vi "Burning.vi"(8 "error in (no error)":errorcluster, 9 "TimeOut(s)":dbl, 10 "burnFilePath":path=path "D:/Project/Tymphany/LT_UpgradeFlash/HDMI Board/LT FW  Files/LT9611 UXC/lt9611uxc_fw.bin", 11 "LT_UpgradeFlash in":refnum<class "LT_UpgradeFlash.lvclass">) -> (0 "error out":errorcluster, 1 "resultStr":string, 2 "ActionResult":bool, 3 "LT_UpgradeFlash out":refnum<class "LT_UpgradeFlash.lvclass">)   [LabVIEW 2017, in "LT_UpgradeFlash.lvclass"]
uses:
  LT_UpgradeFlash.lvclass
  D:/Project/Tymphany/LT_UpgradeFlash/New_Lib/LT_UpgradeFlash_dll/LT_UpgradeFlash_dll/bin/Debug/LT_UpgradeFlash_dll.dll
  New_Lib/LT_UpgradeFlash_dll/LT_UpgradeFlash_dll/bin/Debug/LT_UpgradeFlash_dll.dll
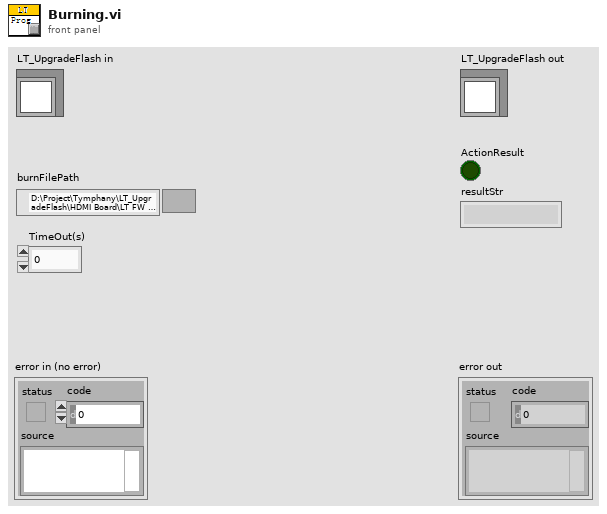
[diagram p1: front panel]
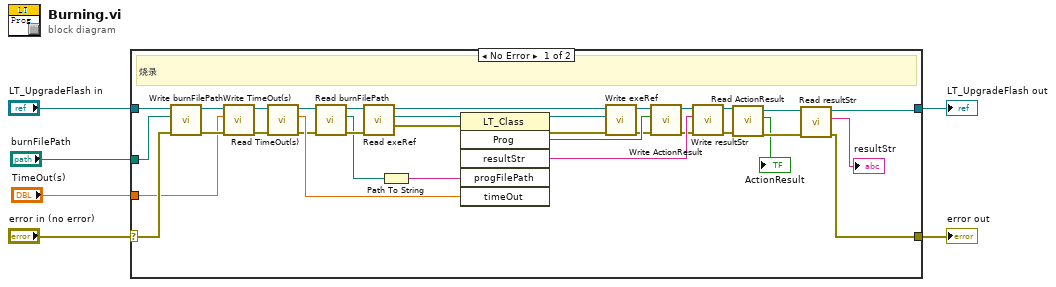
[diagram p0: block diagram]
diagram:
  n1 = case shown="No Error" "error in (no error)" {
    selector: "error in (no error)" -> [w25 w42]
    tunnel: [w17 w42] -> w5
    tunnel: [w18 w41] -> w3
    tunnel: "LT_UpgradeFlash in" -> [w27 w41]
    tunnel: "burnFilePath" -> [w26 _]
    tunnel: "TimeOut(s)" -> [w7 _]
    frame No Error {
      # "烧录"
      n2 = call-dynamic "Write burnFilePath.vi"("error in (no error)"=w25, "burnFilePath"=w26, "LT_UpgradeFlash in"=w27) -> ("error out"=w9:errorcluster, "LT_UpgradeFlash out"=w11:refnum<class "LT_UpgradeFlash.lvclass">)  [unwired: 7 in]
      n3 = call-dynamic "Write TimeOut(s).vi"("error in (no error)"=w9, "TimeOut(s)"=w7, "LT_UpgradeFlash in"=w11) -> ("error out"=w8:errorcluster, "LT_UpgradeFlash out"=w10:refnum<class "LT_UpgradeFlash.lvclass">)  [unwired: 7 in]
      n4 = call-dynamic "Read TimeOut(s).vi"("error in (no error)"=w8, "LT_UpgradeFlash in"=w10) -> ("error out"=w14:errorcluster, "TimeOut(s)"=w38:dbl, "LT_UpgradeFlash out"=w16:refnum<class "LT_UpgradeFlash.lvclass">)  [unwired: 7 in]
      n5 = call-dynamic "Read burnFilePath.vi"("error in (no error)"=w14, "LT_UpgradeFlash in"=w16) -> ("error out"=w13:errorcluster, "burnFilePath"=w12:path, "LT_UpgradeFlash out"=w15:refnum<class "LT_UpgradeFlash.lvclass">)  [unwired: 7 in]
      n6 = call-dynamic "Read exeRef.vi"("error in (no error)"=w13, "LT_UpgradeFlash in"=w15) -> ("error out"=w34:errorcluster, "exeRef"=w40:refnum<k24>, "LT_UpgradeFlash out"=w28:refnum<class "LT_UpgradeFlash.lvclass">)  [unwired: 7 in]
      n7 = Path To String(path=w12) -> (string=w39:string)
      n8 = invoke class="LT_Class" method="Prog"(reference=w40, error in=w34, "progFilePath"=w39, "timeOut"=w38) -> (reference out=w37:refnum<k24>, error out=w33:errorcluster, "Prog"=w36:bool, "resultStr"=w35:string)  [unwired: 2 in, 2 out]
      n9 = call-dynamic "Write exeRef.vi"("error in (no error)"=w33, "exeRef"=w37, "LT_UpgradeFlash in"=w28) -> ("error out"=w31:errorcluster, "LT_UpgradeFlash out"=w32:refnum<class "LT_UpgradeFlash.lvclass">)  [unwired: 7 in]
      n10 = call-dynamic "Write ActionResult.vi"("error in (no error)"=w31, "ActionResult"=w36, "LT_UpgradeFlash in"=w32) -> ("error out"=w29:errorcluster, "LT_UpgradeFlash out"=w30:refnum<class "LT_UpgradeFlash.lvclass">)  [unwired: 7 in]
      n11 = call-dynamic "Write resultStr.vi"("error in (no error)"=w29, "resultStr"=w35, "LT_UpgradeFlash in"=w30) -> ("error out"=w19:errorcluster, "LT_UpgradeFlash out"=w20:refnum<class "LT_UpgradeFlash.lvclass">)  [unwired: 7 in]
      n12 = call-dynamic "Read ActionResult.vi"("error in (no error)"=w19, "LT_UpgradeFlash in"=w20) -> ("error out"=w23:errorcluster, "ActionResult"=→"ActionResult":bool, "LT_UpgradeFlash out"=w24:refnum<class "LT_UpgradeFlash.lvclass">)  [unwired: 7 in]
      n13 = call-dynamic "Read resultStr.vi"("error in (no error)"=w23, "LT_UpgradeFlash in"=w24) -> ("error out"=w17:errorcluster, "resultStr"=→"resultStr":string, "LT_UpgradeFlash out"=w18:refnum<class "LT_UpgradeFlash.lvclass">)  [unwired: 7 in]
    }
    frame Error {
    }
  }
  "error out" <- w5
  "LT_UpgradeFlash out" <- w3
